vi "InAs-GaAs superlattice-111229b- test run.vi"() -> ()   [LabVIEW 2011]
uses:
  development/wait_globals.vi
panel:
  out "Wait Time Remaining(m:s)":string
  out "Waiting":bool
  out "Total Wait Time (m:s)":string
  out "step number  5":i32
  in  "Number of \nGrowth Steps 5":i32=4
  out "step number  4":i32
  in  "Number of \nGrowth Steps 4":i32=4
  out "step number  3":i32
  in  "Number of \nGrowth Steps 3":i32=4
  out "step number  2":i32
  in  "Number of \nGrowth Steps 2":i32=4
  in  "Ga Flow 1":dbl=5.49
  in  "Indium Flow":dbl=45.0
  in  "Number of \nGrowth Steps":i32=4
  out "step number":i32
  in  "As_Gas Flow":dbl=3.4
  in  "Manifold H2 Flow":dbl=730.0
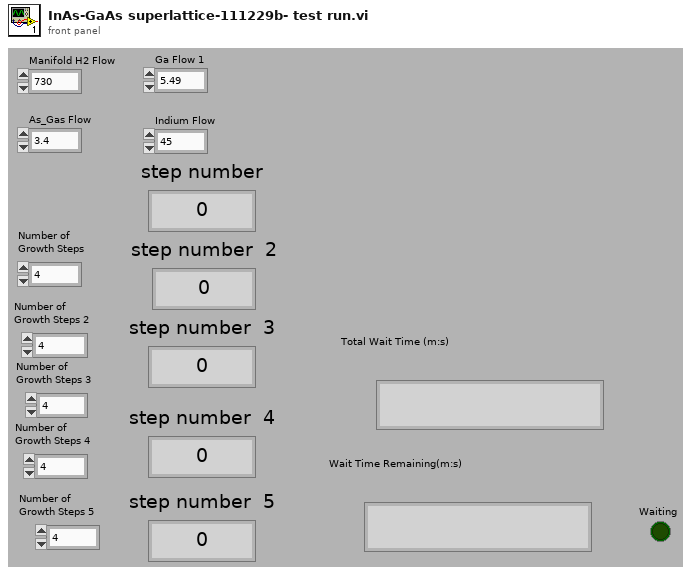
[diagram p1: front panel]
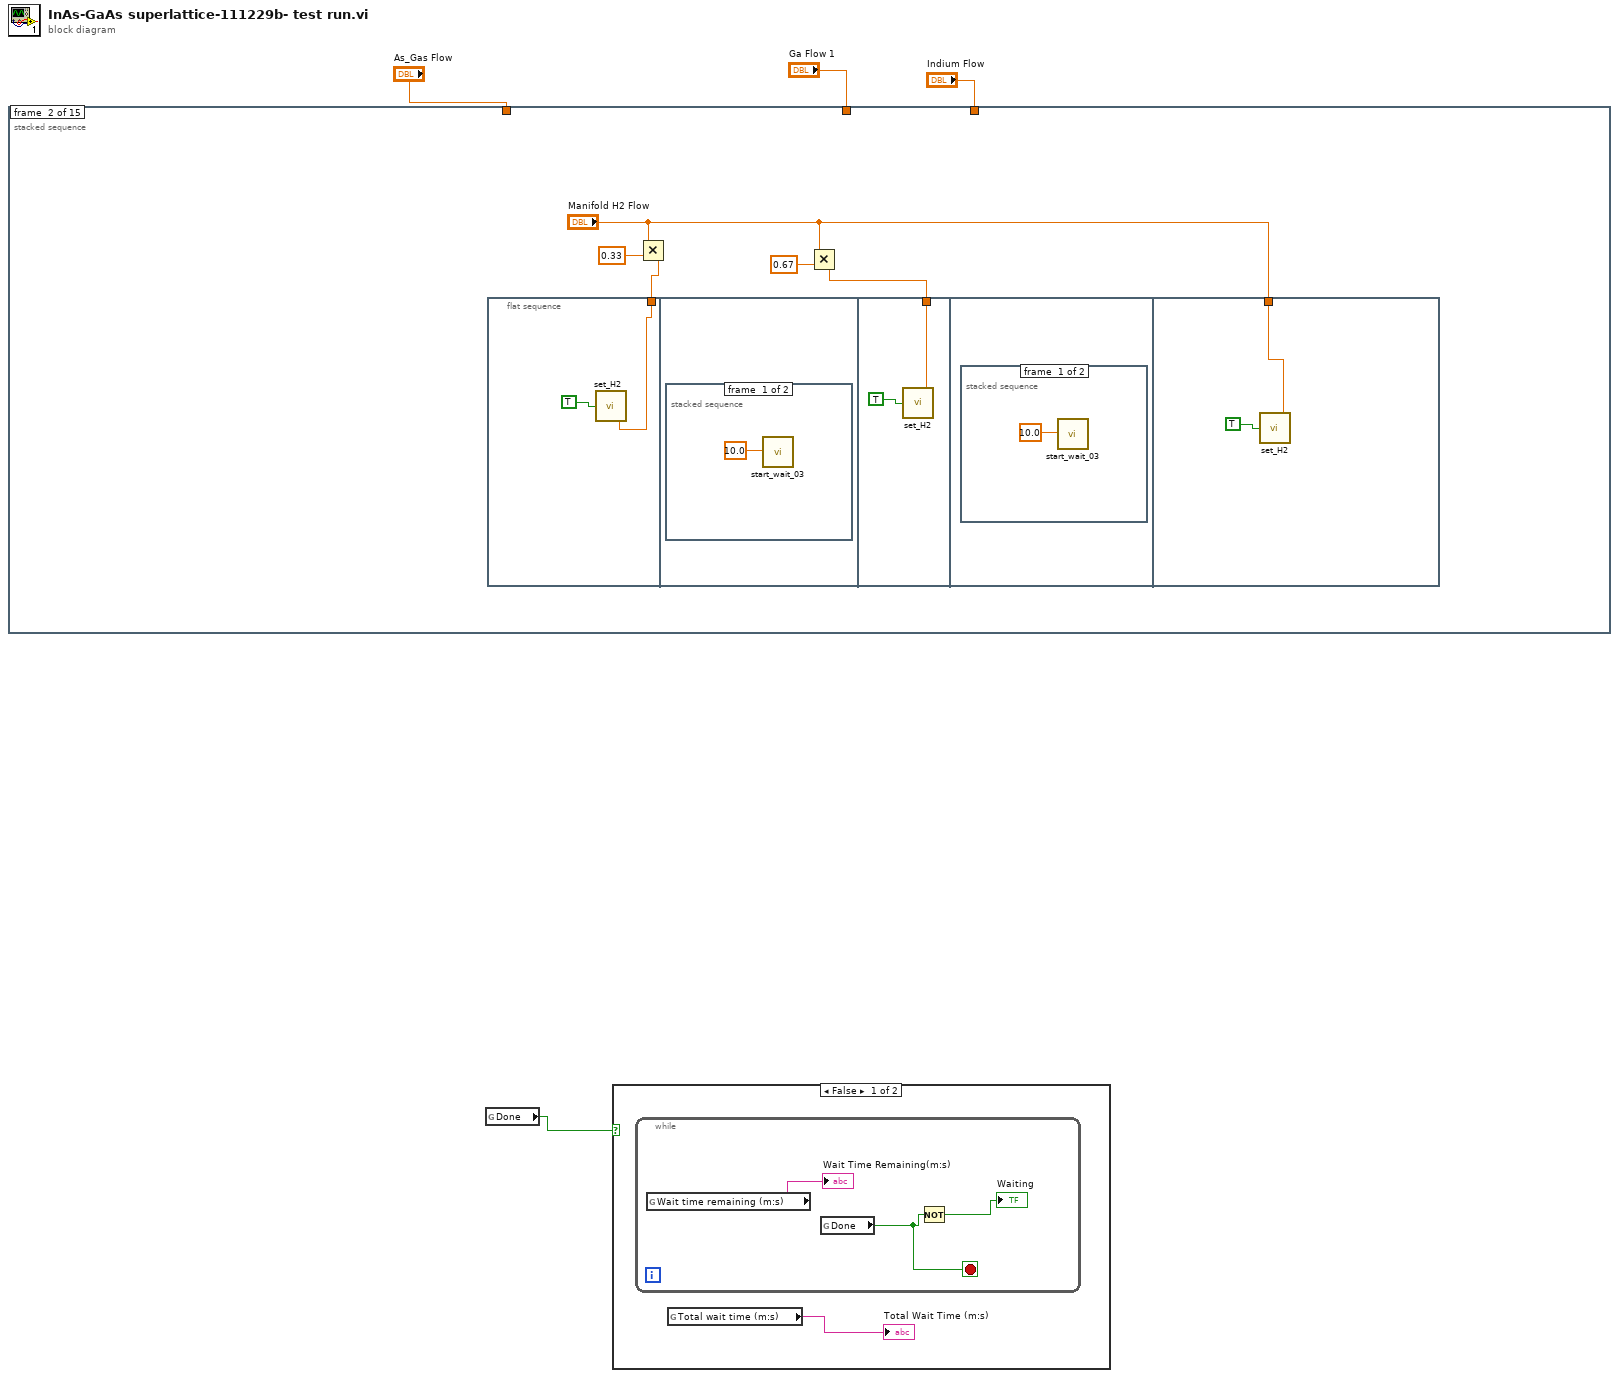
[diagram p0: block diagram]
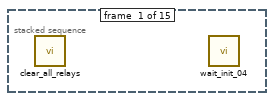
[diagram p3: hidden frame]
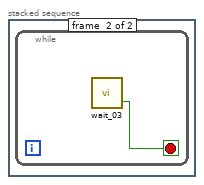
[diagram p4: hidden frame]
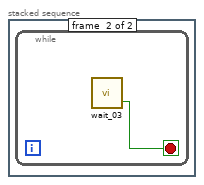
[diagram p5: hidden frame]
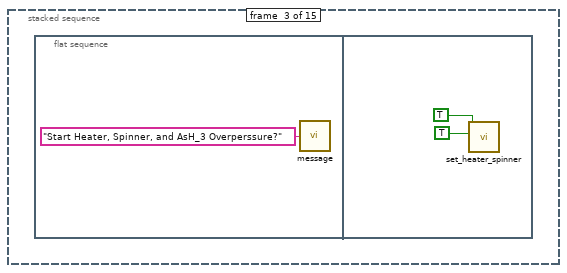
[diagram p6: hidden frame]
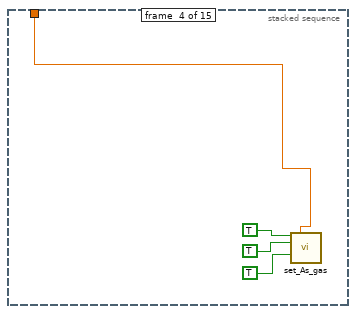
[diagram p7: hidden frame]
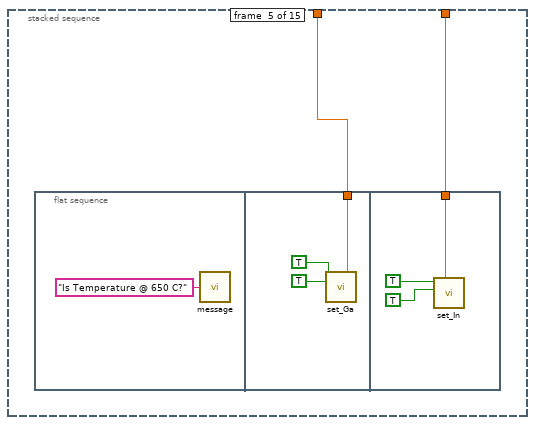
[diagram p8: hidden frame]
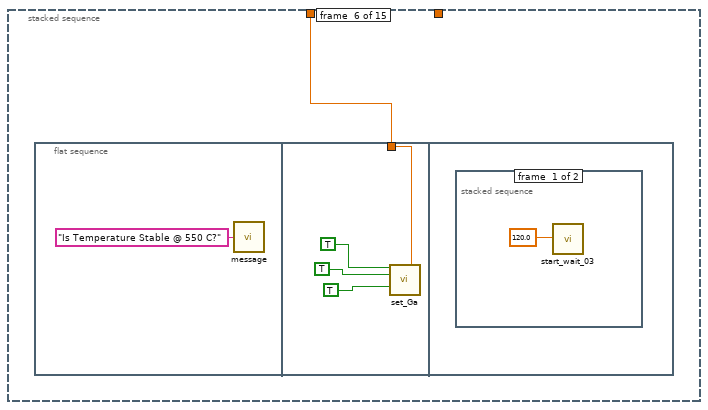
[diagram p9: hidden frame]
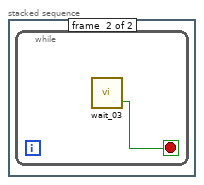
[diagram p10: hidden frame]
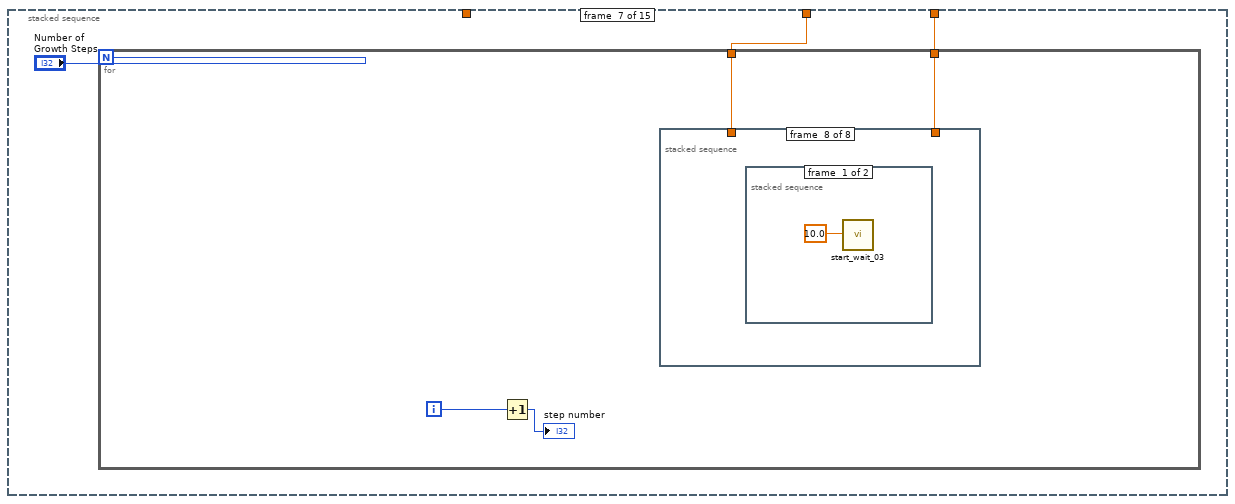
[diagram p11: hidden frame]
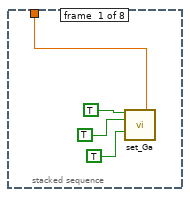
[diagram p12: hidden frame]
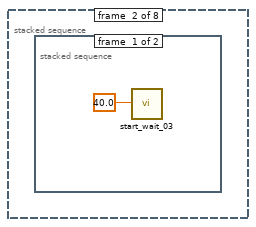
[diagram p13: hidden frame]
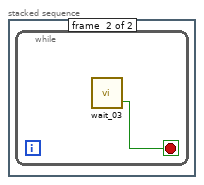
[diagram p14: hidden frame]
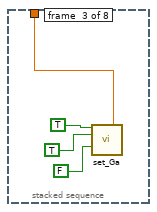
[diagram p15: hidden frame]
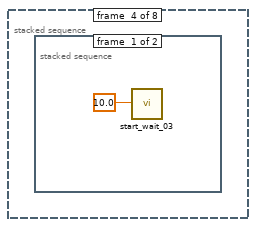
[diagram p16: hidden frame]
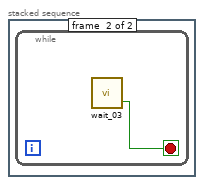
[diagram p17: hidden frame]
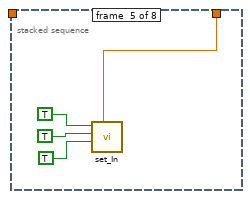
[diagram p18: hidden frame]
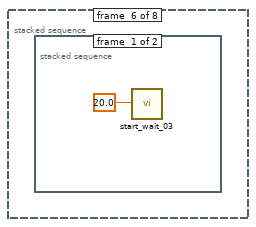
[diagram p19: hidden frame]
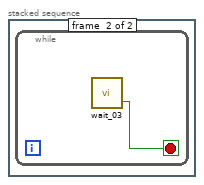
[diagram p20: hidden frame]
diagram:
  n1 = stacked-sequence {
    tunnel: "Ga Flow 1" -> [_ _ _ _ w28 w36 w45 w76 w107 w138 w169 _ _ _ _]
    tunnel: "As_Gas Flow" -> [_ _ _ w23 _ _ _ _ _ _ _ _ _ _ _]
    tunnel: "Indium Flow" -> [_ _ _ _ w27 _ w44 w75 w106 w137 w168 _ _ _ _]
    frame #0 {
      n2 = call "clear_all_relays.vi"() -> ()  [unwired: 2 out]
      n3 = call "wait_init_04.vi"() -> ()  [unwired: 1 in]
    }
    frame #1 {
      n4 = flat-sequence {
        tunnel: w9 -> [w10]
        tunnel: w7 -> [w14]
        tunnel: "Manifold H2 Flow" -> [w18]
        frame #0 {
          n5 = call "set_H2.vi"("Manifold H2 Flow"=w10, "H2 Active"=TRUE) -> ()  [unwired: 2 in, 2 out]
        }
        frame #1 {
          n6 = stacked-sequence {
            frame #0 {
              n7 = call "start_wait_03.vi"("Total wait time (s)"=10.0 ("Wait (s)")) -> ()
            }
            frame #1 {
              n8 = while {
                stop <- w13 stop-if-true
                n9 = call "wait_03.vi"() -> ("Done"=w13:bool)  [unwired: 1 in, 1 out]
              }
            }
          }
        }
        frame #2 {
          n10 = call "set_H2.vi"("Manifold H2 Flow"=w14, "H2 Active"=TRUE) -> ()  [unwired: 2 in, 2 out]
        }
        frame #3 {
          n11 = stacked-sequence {
            frame #0 {
              n12 = call "start_wait_03.vi"("Total wait time (s)"=10.0 ("Wait (s)")) -> ()
            }
            frame #1 {
              n13 = while {
                stop <- w17 stop-if-true
                n14 = call "wait_03.vi"() -> ("Done"=w17:bool)  [unwired: 1 in, 1 out]
              }
            }
          }
        }
        frame #4 {
          n15 = call "set_H2.vi"("Manifold H2 Flow"=w18, "H2 Active"=TRUE) -> ()  [unwired: 2 in, 2 out]
        }
      }
      n16 = Multiply(x="Manifold H2 Flow", y=0.33) -> (x*y=w9:dbl)
      n17 = Multiply(x="Manifold H2 Flow", y=0.67) -> (x*y=w7:dbl)
    }
    frame #2 {
      n18 = flat-sequence {
        frame #0 {
          n19 = call "message.vi"("message"="Start Heater, Spinner, and AsH_3 Overperssure?") -> ()
        }
        frame #1 {
          n20 = call "set_heater_spinner.vi"("Spinner"=TRUE, "Heater"=TRUE) -> ()  [unwired: 1 in, 7 out]
        }
      }
    }
    frame #3 {
      n21 = call "set_As_gas.vi"("As_Gas Active"=TRUE, "As_Gas Flow"=w23, "As_Gas In"=TRUE, "As_Gas Run"=TRUE) -> ()  [unwired: 2 in, 10 out]
    }
    frame #4 {
      n22 = flat-sequence {
        tunnel: w28 -> [w30]
        tunnel: w27 -> [w33]
        frame #0 {
          n23 = call "message.vi"("message"="Is Temperature @ 650 C?") -> ()
        }
        frame #1 {
          n24 = call "set_Ga.vi"("Ga Active"=TRUE, "Ga Flow 1"=w30, "Ga Bubbler"=TRUE) -> ()  [unwired: 5 in, 8 out]
        }
        frame #2 {
          n25 = call "set_In.vi"("Indium Flow"=w33, "In Bubbler"=TRUE ("Ga Bubbler"), "In Active"=TRUE ("Ga Active")) -> ()  [unwired: 2 in, 5 out]
        }
      }
    }
    frame #5 {
      n26 = flat-sequence {
        tunnel: w36 -> [w38]
        frame #0 {
          n27 = call "message.vi"("message"="Is Temperature Stable @ 550 C?") -> ()
        }
        frame #1 {
          n28 = call "set_Ga.vi"("Ga Active"=TRUE ("P_Gas Active"), "Ga Flow 1"=w38, "Ga Bubbler"=TRUE ("P_Gas In"), "Ga Run"=TRUE ("P_Gas Run")) -> ()  [unwired: 4 in, 8 out]
        }
        frame #2 {
          n29 = stacked-sequence {
            frame #0 {
              n30 = call "start_wait_03.vi"("Total wait time (s)"=120.0 ("Wait (s)")) -> ()
            }
            frame #1 {
              n31 = while {
                stop <- w43 stop-if-true
                n32 = call "wait_03.vi"() -> ("Done"=w43:bool)  [unwired: 1 in, 1 out]
              }
            }
          }
        }
      }
    }
    frame #6 {
      n33 = for {
        N: "Number of \nGrowth Steps" -> [_]
        tunnel: w45 -> [w48]
        tunnel: w44 -> [w47]
        i -> [w49]
        n34 = Increment(x=w49) -> (x+1=→"step number":i32)
        n35 = stacked-sequence {
          tunnel: w47 -> [_ _ _ _ w63 _ w70 _]
          tunnel: w48 -> [w51 _ w57 _ _ _ _ _]
          frame #0 {
            n36 = call "set_Ga.vi"("Ga Active"=TRUE ("P_Gas Active"), "Ga Flow 1"=w51, "Ga Bubbler"=TRUE ("P_Gas In"), "Ga Run"=TRUE ("P_Gas Run")) -> ()  [unwired: 4 in, 8 out]
          }
          frame #1 {
            n37 = stacked-sequence {
              frame #0 {
                n38 = call "start_wait_03.vi"("Total wait time (s)"=40.0 ("Wait (s)")) -> ()
              }
              frame #1 {
                n39 = while {
                  stop <- w56 stop-if-true
                  n40 = call "wait_03.vi"() -> ("Done"=w56:bool)  [unwired: 1 in, 1 out]
                }
              }
            }
          }
          frame #2 {
            n41 = call "set_Ga.vi"("Ga Active"=TRUE ("P_Gas Active"), "Ga Flow 1"=w57, "Ga Bubbler"=TRUE ("P_Gas In"), "Ga Run"=FALSE ("P_Gas Run")) -> ()  [unwired: 4 in, 8 out]
          }
          frame #3 {
            n42 = stacked-sequence {
              frame #0 {
                n43 = call "start_wait_03.vi"("Total wait time (s)"=10.0 ("Wait (s)")) -> ()
              }
              frame #1 {
                n44 = while {
                  stop <- w62 stop-if-true
                  n45 = call "wait_03.vi"() -> ("Done"=w62:bool)  [unwired: 1 in, 1 out]
                }
              }
            }
          }
          frame #4 {
            n46 = call "set_In.vi"("Indium Flow"=w63, "In Run"=TRUE ("P_Gas Run"), "In Bubbler"=TRUE ("P_Gas In"), "In Active"=TRUE ("P_Gas Active")) -> ()  [unwired: 1 in, 5 out]
          }
          frame #5 {
            n47 = stacked-sequence {
              frame #0 {
                n48 = call "start_wait_03.vi"("Total wait time (s)"=20.0 ("Wait (s)")) -> ()
              }
              frame #1 {
                n49 = while {
                  stop <- w68 stop-if-true
                  n50 = call "wait_03.vi"() -> ("Done"=w68:bool)  [unwired: 1 in, 1 out]
                }
              }
            }
          }
          frame #6 {
            n51 = call "set_In.vi"("Indium Flow"=w70, "In Run"=FALSE ("P_Gas Run"), "In Bubbler"=TRUE ("P_Gas In"), "In Active"=TRUE ("P_Gas Active")) -> ()  [unwired: 1 in, 5 out]
          }
          frame #7 {
            n52 = stacked-sequence {
              frame #0 {
                n53 = call "start_wait_03.vi"("Total wait time (s)"=10.0 ("Wait (s)")) -> ()
              }
              frame #1 {
                n54 = while {
                  stop <- w74 stop-if-true
                  n55 = call "wait_03.vi"() -> ("Done"=w74:bool)  [unwired: 1 in, 1 out]
                }
              }
            }
          }
        }
      }
    }
    frame #7 {
      n56 = for {
        N: "Number of \nGrowth Steps 2" -> [_]
        tunnel: w76 -> [w79]
        tunnel: w75 -> [w78]
        i -> [w80]
        n57 = Increment(x=w80) -> (x+1=→"step number  2":i32)
        n58 = stacked-sequence {
          tunnel: w78 -> [_ _ _ _ w94 _ w101 _]
          tunnel: w79 -> [w82 _ w88 _ _ _ _ _]
          frame #0 {
            n59 = call "set_Ga.vi"("Ga Active"=TRUE ("P_Gas Active"), "Ga Flow 1"=w82, "Ga Bubbler"=TRUE ("P_Gas In"), "Ga Run"=TRUE ("P_Gas Run")) -> ()  [unwired: 4 in, 8 out]
          }
          frame #1 {
            n60 = stacked-sequence {
              frame #0 {
                n61 = call "start_wait_03.vi"("Total wait time (s)"=40.0 ("Wait (s)")) -> ()
              }
              frame #1 {
                n62 = while {
                  stop <- w87 stop-if-true
                  n63 = call "wait_03.vi"() -> ("Done"=w87:bool)  [unwired: 1 in, 1 out]
                }
              }
            }
          }
          frame #2 {
            n64 = call "set_Ga.vi"("Ga Active"=TRUE ("P_Gas Active"), "Ga Flow 1"=w88, "Ga Bubbler"=TRUE ("P_Gas In"), "Ga Run"=FALSE ("P_Gas Run")) -> ()  [unwired: 4 in, 8 out]
          }
          frame #3 {
            n65 = stacked-sequence {
              frame #0 {
                n66 = call "start_wait_03.vi"("Total wait time (s)"=10.0 ("Wait (s)")) -> ()
              }
              frame #1 {
                n67 = while {
                  stop <- w93 stop-if-true
                  n68 = call "wait_03.vi"() -> ("Done"=w93:bool)  [unwired: 1 in, 1 out]
                }
              }
            }
          }
          frame #4 {
            n69 = call "set_In.vi"("Indium Flow"=w94, "In Run"=TRUE ("P_Gas Run"), "In Bubbler"=TRUE ("P_Gas In"), "In Active"=TRUE ("P_Gas Active")) -> ()  [unwired: 1 in, 5 out]
          }
          frame #5 {
            n70 = stacked-sequence {
              frame #0 {
                n71 = call "start_wait_03.vi"("Total wait time (s)"=20.0 ("Wait (s)")) -> ()
              }
              frame #1 {
                n72 = while {
                  stop <- w99 stop-if-true
                  n73 = call "wait_03.vi"() -> ("Done"=w99:bool)  [unwired: 1 in, 1 out]
                }
              }
            }
          }
          frame #6 {
            n74 = call "set_In.vi"("Indium Flow"=w101, "In Run"=FALSE ("P_Gas Run"), "In Bubbler"=TRUE ("P_Gas In"), "In Active"=TRUE ("P_Gas Active")) -> ()  [unwired: 1 in, 5 out]
          }
          frame #7 {
            n75 = stacked-sequence {
              frame #0 {
                n76 = call "start_wait_03.vi"("Total wait time (s)"=20.0 ("Wait (s)")) -> ()
              }
              frame #1 {
                n77 = while {
                  stop <- w105 stop-if-true
                  n78 = call "wait_03.vi"() -> ("Done"=w105:bool)  [unwired: 1 in, 1 out]
                }
              }
            }
          }
        }
      }
    }
    frame #8 {
      n79 = for {
        N: "Number of \nGrowth Steps 3" -> [_]
        tunnel: w107 -> [w110]
        tunnel: w106 -> [w109]
        i -> [w111]
        n80 = Increment(x=w111) -> (x+1=→"step number  3":i32)
        n81 = stacked-sequence {
          tunnel: w109 -> [_ _ _ _ w125 _ w132 _]
          tunnel: w110 -> [w113 _ w119 _ _ _ _ _]
          frame #0 {
            n82 = call "set_Ga.vi"("Ga Active"=TRUE ("P_Gas Active"), "Ga Flow 1"=w113, "Ga Bubbler"=TRUE ("P_Gas In"), "Ga Run"=TRUE ("P_Gas Run")) -> ()  [unwired: 4 in, 8 out]
          }
          frame #1 {
            n83 = stacked-sequence {
              frame #0 {
                n84 = call "start_wait_03.vi"("Total wait time (s)"=40.0 ("Wait (s)")) -> ()
              }
              frame #1 {
                n85 = while {
                  stop <- w118 stop-if-true
                  n86 = call "wait_03.vi"() -> ("Done"=w118:bool)  [unwired: 1 in, 1 out]
                }
              }
            }
          }
          frame #2 {
            n87 = call "set_Ga.vi"("Ga Active"=TRUE ("P_Gas Active"), "Ga Flow 1"=w119, "Ga Bubbler"=TRUE ("P_Gas In"), "Ga Run"=FALSE ("P_Gas Run")) -> ()  [unwired: 4 in, 8 out]
          }
          frame #3 {
            n88 = stacked-sequence {
              frame #0 {
                n89 = call "start_wait_03.vi"("Total wait time (s)"=10.0 ("Wait (s)")) -> ()
              }
              frame #1 {
                n90 = while {
                  stop <- w124 stop-if-true
                  n91 = call "wait_03.vi"() -> ("Done"=w124:bool)  [unwired: 1 in, 1 out]
                }
              }
            }
          }
          frame #4 {
            n92 = call "set_In.vi"("Indium Flow"=w125, "In Run"=TRUE ("P_Gas Run"), "In Bubbler"=TRUE ("P_Gas In"), "In Active"=TRUE ("P_Gas Active")) -> ()  [unwired: 1 in, 5 out]
          }
          frame #5 {
            n93 = stacked-sequence {
              frame #0 {
                n94 = call "start_wait_03.vi"("Total wait time (s)"=20.0 ("Wait (s)")) -> ()
              }
              frame #1 {
                n95 = while {
                  stop <- w130 stop-if-true
                  n96 = call "wait_03.vi"() -> ("Done"=w130:bool)  [unwired: 1 in, 1 out]
                }
              }
            }
          }
          frame #6 {
            n97 = call "set_In.vi"("Indium Flow"=w132, "In Run"=FALSE ("P_Gas Run"), "In Bubbler"=TRUE ("P_Gas In"), "In Active"=TRUE ("P_Gas Active")) -> ()  [unwired: 1 in, 5 out]
          }
          frame #7 {
            n98 = stacked-sequence {
              frame #0 {
                n99 = call "start_wait_03.vi"("Total wait time (s)"=30.0 ("Wait (s)")) -> ()
              }
              frame #1 {
                n100 = while {
                  stop <- w136 stop-if-true
                  n101 = call "wait_03.vi"() -> ("Done"=w136:bool)  [unwired: 1 in, 1 out]
                }
              }
            }
          }
        }
      }
    }
    frame #9 {
      n102 = for {
        N: "Number of \nGrowth Steps 4" -> [_]
        tunnel: w138 -> [w141]
        tunnel: w137 -> [w140]
        i -> [w142]
        n103 = Increment(x=w142) -> (x+1=→"step number  4":i32)
        n104 = stacked-sequence {
          tunnel: w140 -> [_ _ _ _ w156 _ w163 _]
          tunnel: w141 -> [w144 _ w150 _ _ _ _ _]
          frame #0 {
            n105 = call "set_Ga.vi"("Ga Active"=TRUE ("P_Gas Active"), "Ga Flow 1"=w144, "Ga Bubbler"=TRUE ("P_Gas In"), "Ga Run"=TRUE ("P_Gas Run")) -> ()  [unwired: 4 in, 8 out]
          }
          frame #1 {
            n106 = stacked-sequence {
              frame #0 {
                n107 = call "start_wait_03.vi"("Total wait time (s)"=40.0 ("Wait (s)")) -> ()
              }
              frame #1 {
                n108 = while {
                  stop <- w149 stop-if-true
                  n109 = call "wait_03.vi"() -> ("Done"=w149:bool)  [unwired: 1 in, 1 out]
                }
              }
            }
          }
          frame #2 {
            n110 = call "set_Ga.vi"("Ga Active"=TRUE ("P_Gas Active"), "Ga Flow 1"=w150, "Ga Bubbler"=TRUE ("P_Gas In"), "Ga Run"=FALSE ("P_Gas Run")) -> ()  [unwired: 4 in, 8 out]
          }
          frame #3 {
            n111 = stacked-sequence {
              frame #0 {
                n112 = call "start_wait_03.vi"("Total wait time (s)"=10.0 ("Wait (s)")) -> ()
              }
              frame #1 {
                n113 = while {
                  stop <- w155 stop-if-true
                  n114 = call "wait_03.vi"() -> ("Done"=w155:bool)  [unwired: 1 in, 1 out]
                }
              }
            }
          }
          frame #4 {
            n115 = call "set_In.vi"("Indium Flow"=w156, "In Run"=TRUE ("P_Gas Run"), "In Bubbler"=TRUE ("P_Gas In"), "In Active"=TRUE ("P_Gas Active")) -> ()  [unwired: 1 in, 5 out]
          }
          frame #5 {
            n116 = stacked-sequence {
              frame #0 {
                n117 = call "start_wait_03.vi"("Total wait time (s)"=20.0 ("Wait (s)")) -> ()
              }
              frame #1 {
                n118 = while {
                  stop <- w161 stop-if-true
                  n119 = call "wait_03.vi"() -> ("Done"=w161:bool)  [unwired: 1 in, 1 out]
                }
              }
            }
          }
          frame #6 {
            n120 = call "set_In.vi"("Indium Flow"=w163, "In Run"=FALSE ("P_Gas Run"), "In Bubbler"=TRUE ("P_Gas In"), "In Active"=TRUE ("P_Gas Active")) -> ()  [unwired: 1 in, 5 out]
          }
          frame #7 {
            n121 = stacked-sequence {
              frame #0 {
                n122 = call "start_wait_03.vi"("Total wait time (s)"=45.0 ("Wait (s)")) -> ()
              }
              frame #1 {
                n123 = while {
                  stop <- w167 stop-if-true
                  n124 = call "wait_03.vi"() -> ("Done"=w167:bool)  [unwired: 1 in, 1 out]
                }
              }
            }
          }
        }
      }
    }
    frame #10 {
      n125 = for {
        N: "Number of \nGrowth Steps 5" -> [_]
        tunnel: w169 -> [w171]
        tunnel: w168 -> [w172]
        i -> [w173]
        n126 = Increment(x=w173) -> (x+1=→"step number  5":i32)
        n127 = stacked-sequence {
          tunnel: w172 -> [_ _ _ _ w187 _ w194 _]
          tunnel: [_ _ _ _ _ _ w194 _] -> _
          tunnel: w171 -> [w175 _ w181 _ _ _ _ _]
          frame #0 {
            n128 = call "set_Ga.vi"("Ga Active"=TRUE ("P_Gas Active"), "Ga Flow 1"=w175, "Ga Bubbler"=TRUE ("P_Gas In"), "Ga Run"=TRUE ("P_Gas Run")) -> ()  [unwired: 4 in, 8 out]
          }
          frame #1 {
            n129 = stacked-sequence {
              frame #0 {
                n130 = call "start_wait_03.vi"("Total wait time (s)"=40.0 ("Wait (s)")) -> ()
              }
              frame #1 {
                n131 = while {
                  stop <- w180 stop-if-true
                  n132 = call "wait_03.vi"() -> ("Done"=w180:bool)  [unwired: 1 in, 1 out]
                }
              }
            }
          }
          frame #2 {
            n133 = call "set_Ga.vi"("Ga Active"=TRUE ("P_Gas Active"), "Ga Flow 1"=w181, "Ga Bubbler"=TRUE ("P_Gas In"), "Ga Run"=FALSE ("P_Gas Run")) -> ()  [unwired: 4 in, 8 out]
          }
          frame #3 {
            n134 = stacked-sequence {
              frame #0 {
                n135 = call "start_wait_03.vi"("Total wait time (s)"=10.0 ("Wait (s)")) -> ()
              }
              frame #1 {
                n136 = while {
                  stop <- w186 stop-if-true
                  n137 = call "wait_03.vi"() -> ("Done"=w186:bool)  [unwired: 1 in, 1 out]
                }
              }
            }
          }
          frame #4 {
            n138 = call "set_In.vi"("Indium Flow"=w187, "In Run"=TRUE ("P_Gas Run"), "In Bubbler"=TRUE ("P_Gas In"), "In Active"=TRUE ("P_Gas Active")) -> ()  [unwired: 1 in, 5 out]
          }
          frame #5 {
            n139 = stacked-sequence {
              frame #0 {
                n140 = call "start_wait_03.vi"("Total wait time (s)"=20.0 ("Wait (s)")) -> ()
              }
              frame #1 {
                n141 = while {
                  stop <- w192 stop-if-true
                  n142 = call "wait_03.vi"() -> ("Done"=w192:bool)  [unwired: 1 in, 1 out]
                }
              }
            }
          }
          frame #6 {
            n143 = call "set_In.vi"("Indium Flow"=w194, "In Run"=FALSE ("P_Gas Run"), "In Bubbler"=TRUE ("P_Gas In"), "In Active"=TRUE ("P_Gas Active")) -> ()  [unwired: 1 in, 5 out]
          }
          frame #7 {
            n144 = stacked-sequence {
              frame #0 {
                n145 = call "start_wait_03.vi"("Total wait time (s)"=60.0 ("Wait (s)")) -> ()
              }
              frame #1 {
                n146 = while {
                  stop <- w198 stop-if-true
                  n147 = call "wait_03.vi"() -> ("Done"=w198:bool)  [unwired: 1 in, 1 out]
                }
              }
            }
          }
        }
      }
    }
    frame #11 {
      n148 = flat-sequence {
        frame #0 {
          n149 = call "set_heater_spinner.vi"("Spinner"=TRUE ("Ga Active")) -> ()  [unwired: 2 in, 7 out]
        }
        frame #1 {
          n150 = call "set_Ga.vi"("Ga Active"=TRUE, "Ga Flow 1"=10.0) -> ()  [unwired: 6 in, 8 out]
        }
        frame #2 {
          n151 = call "set_In.vi"("Indium Flow"=100.0 ("Aluminum Flow"), "In Active"=TRUE ("Ga Active")) -> ()  [unwired: 3 in, 5 out]
        }
        frame #3 {
          n152 = stacked-sequence {
            frame #0 {
              n153 = call "start_wait_03.vi"("Total wait time (s)"=20.0 ("Wait (s)")) -> ()
            }
            frame #1 {
              n154 = while {
                stop <- w205 stop-if-true
                n155 = call "wait_03.vi"() -> ("Done"=w205:bool)  [unwired: 1 in, 1 out]
              }
            }
          }
        }
      }
    }
    frame #12 {
      n156 = flat-sequence {
        frame #0 {
          n157 = call "set_Ga.vi"("Ga Remote"=FALSE) -> ()  [unwired: 7 in, 8 out]
        }
        frame #1 {
          n158 = call "set_In.vi"("In Run"=FALSE ("Ga Remote")) -> ()  [unwired: 4 in, 5 out]
        }
        frame #2 {
          n159 = call "message.vi"("message"="Is Temperature < 300C?") -> ()
        }
      }
    }
    frame #13 {
      n160 = call "set_As_gas.vi"("As_Gas Remote"=FALSE) -> ()  [unwired: 5 in, 10 out]
    }
    frame #14 {
      n161 = flat-sequence {
        frame #0 {
          n162 = call "message.vi"("message"="Is Temperarure < 100C?") -> ()
        }
        frame #1 {
          n163 = call "set_heater_spinner.vi"("Heater/Spinner Remote"=FALSE) -> ()  [unwired: 2 in, 7 out]
        }
        frame #2 {
          n164 = call "set_H2.vi"("H2N2 Remote"=FALSE) -> ()  [unwired: 3 in, 2 out]
        }
      }
    }
  }
  n165 = global read "wait_globals.vi" "Done"() -> (w1:bool)
  n166 = case shown="False" w1 {
    frame False {
      n167 = global read "wait_globals.vi" "Total wait time (m:s)"() -> (→"Total Wait Time (m:s)":string)
    }
    frame True {
    }
  }
  n168 = while {
    stop <- w214 stop-if-true
    n169 = global read "wait_globals.vi" "Wait time remaining (m:s)"() -> (→"Wait Time Remaining(m:s)":string)
    n170 = global read "wait_globals.vi" "Done"() -> (w214:bool)
    n171 = Not(x=w214) -> (.not. x?=→"Waiting":bool)
  }
